vi "All Services.vi"(8 "error in (no error)":errorcluster, 11 "Values in":refnum<class "Values.lvclass">) -> (0 "error out":errorcluster, 2 "All Services":refnum<class "Service.lvclass">[](array[class]), 3 "Values out":refnum<class "Values.lvclass">)   [LabVIEW 2020, in "HTTP Server.lvlib" / "Values.lvclass"]
uses:
  Values.lvclass
  Service/Service.lvclass
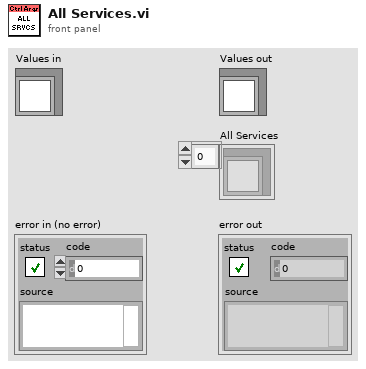
[diagram p1: front panel]
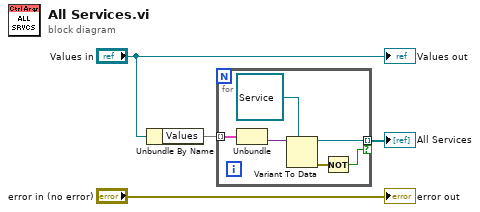
[diagram p0: block diagram]
diagram:
  n1 = Unbundle By Name("Values in") -> ("Values"=w2:map{string, variant})
  n2 = for {
    tunnel: w2 -> [w10] mode=indexing
    tunnel: [w7] -> w1 mode=indexing if=w5
    n3 = Unbundle(w10) -> ("Argument"=w9:variant)  [unwired: 1 out]
    n4 = Variant To Data(type=refnum<class "Service.lvclass"> refnum ("HTTP Server.lvlib:Service.lvclass"), Variant=w9) -> (data=w7:refnum<class "Service.lvclass">, error out=w6:errorcluster)  [unwired: 1 in]
    n5 = Not(x=w6) -> (.not. x?=w5:bool)
  }
  "All Services" <- w1
  "error out" <- "error in (no error)"
  "Values out" <- "Values in"
